vi "ta_calc_diff.vi"(0 "data in":dbl[][](array[numeric]), 5 "anisotropy input":T1, 9 "ref in":dbl[][](array[numeric]), 11 "Algorithm":T2=3 items=["<(S*-S)/S>/ln(10)", "<S*/S>-1", "<S*/PD*>/<S/PD>", "<S*/Sref*>/<S/Sref>", "<S*/Sref*/PD*>/<S/Sref>", "<S*/Sref*>/<S/Sref>_alt", "MA/r", "MA/r Sagnac", "FROG"], 12 "PD values in":dbl[][](array[numeric])) -> (1 "pumped std":dbl[](array[numeric]), 2 "anisotropy":T1, 3 "unpumped std":dbl[](array[numeric]), 4 "pumped":dbl[](array[numeric]), 6 "unpumped":dbl[](array[numeric]), 8 "diff std":dbl[](array[numeric]), 10 "diff":dbl[](array[numeric]), 14 "ref std":dbl[](array[numeric]), 15 "ref mean":dbl[](array[numeric]))   [LabVIEW 2019]
uses:
  data_algorithm.ctl
  <vilib>/Analysis/baseanly.llb/Mean (DBL).vi
  <vilib>/Analysis/NI_AALBase.lvlib
panel:
  out "size data":i32[](array[numeric])
  out "size ref":i32[](array[numeric])
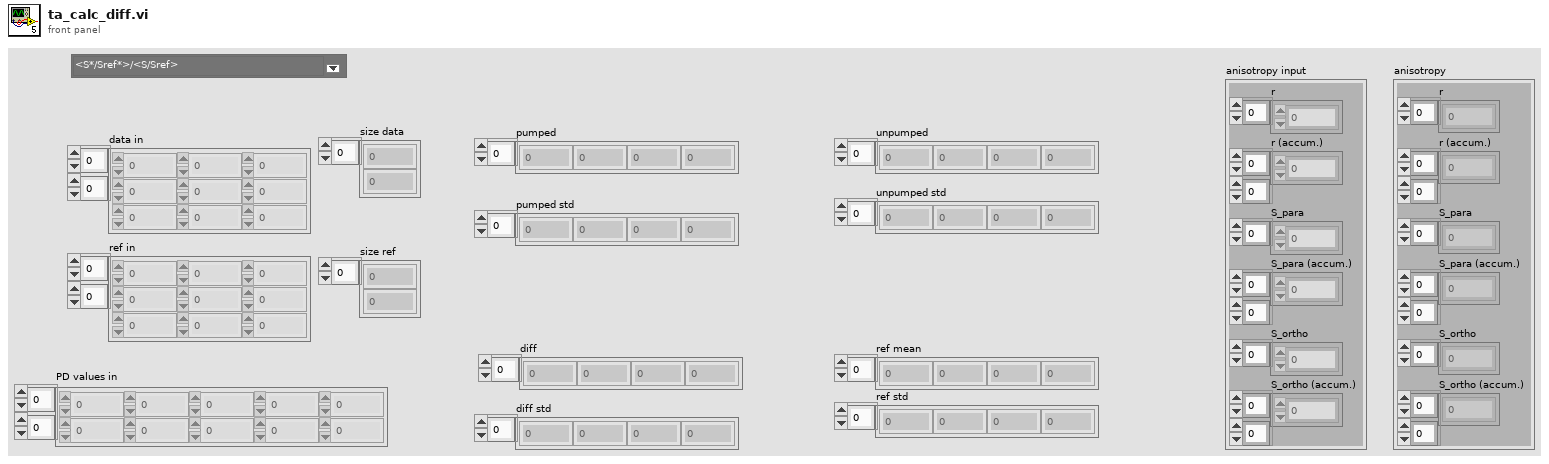
[diagram p1: front panel]
types:
  T1 = cluster{"r":dbl[], "r (accum.)":dbl[][], "S_para":dbl[], "S_para (accum.)":dbl[][], "S_ortho":dbl[], "S_ortho (accum.)":dbl[][]}
  T2 = typedef "data_algorithm.ctl" = u16
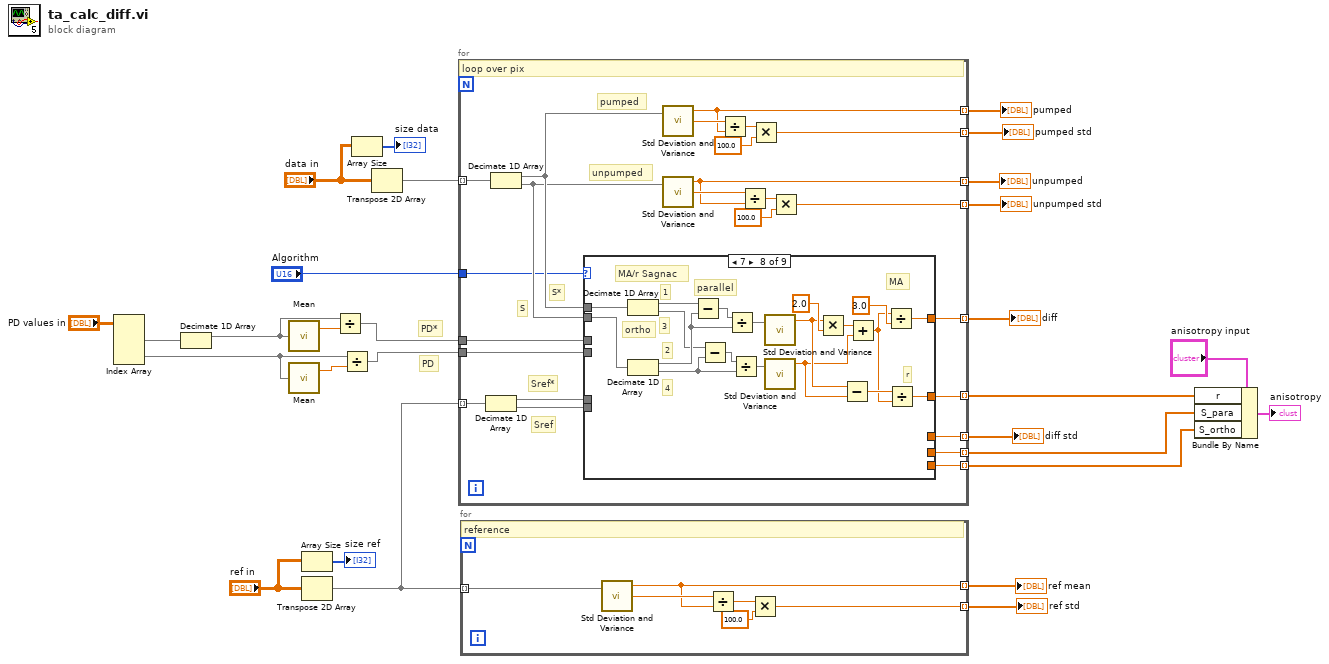
[diagram p0: block diagram]
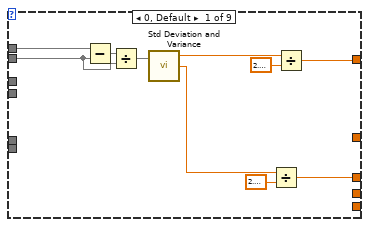
[diagram p2: hidden frame]
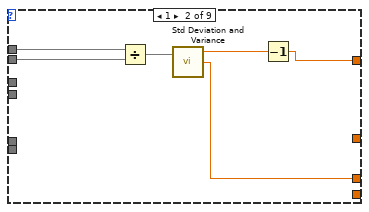
[diagram p3: hidden frame]
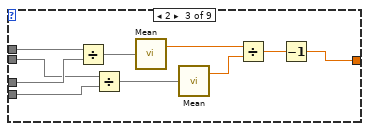
[diagram p4: hidden frame]
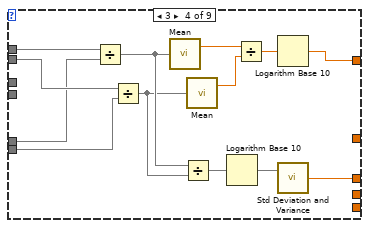
[diagram p5: hidden frame]
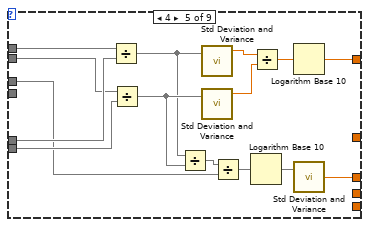
[diagram p6: hidden frame]
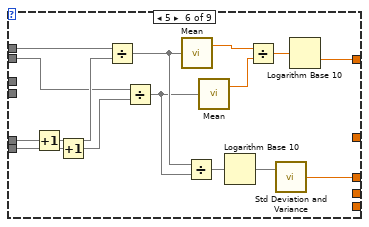
[diagram p7: hidden frame]
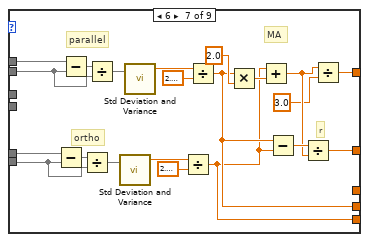
[diagram p8: hidden frame]
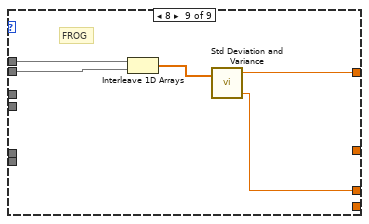
[diagram p9: hidden frame]
diagram:
  # "PD"
  # "PD*"
  n1 = Index Array(array="PD values in") -> (element #1=w8:dbl[], element #2=w11:dbl[])  [unwired: 4 in]
  n2 = Decimate 1D Array(w8) -> (w7:dbl[])  [unwired: 1 out]
  n3 = call-poly <vilib>:"Mean.vi"("X"=w7) -> ("mean"=w12:dbl)  [unwired: 1 out]
  n4 = call-poly <vilib>:"Mean.vi"("X"=w11) -> ("mean"=w10:dbl)  [unwired: 1 out]
  n5 = Array Size(array="ref in") -> (size(s)=→"size ref":i32[])
  n6 = Transpose 2D Array(2D array="ref in") -> (transposed array=w16:dbl[][])
  n7 = Divide(x=w7, y=w12) -> (x/y=w13:dbl[])
  n8 = Divide(x=w11, y=w10) -> (x/y=w9:dbl[])
  n9 = Array Size(array="data in") -> (size(s)=→"size data":i32[])
  n10 = Transpose 2D Array(2D array="data in") -> (transposed array=w22:dbl[][])
  n11 = for {
    tunnel: w22 -> [w50] mode=indexing
    tunnel: [w41] -> w28 mode=indexing
    tunnel: [w48] -> w27 mode=indexing
    tunnel: [w45] -> w20 mode=indexing
    tunnel: [w40] -> w19 mode=indexing
    tunnel: "Algorithm" -> [w39]
    tunnel: [w38] -> w17 mode=indexing
    tunnel: w13 -> [w33]
    tunnel: w9 -> [w37]
    tunnel: w16 -> [w36] mode=indexing
    tunnel: [w32] -> w6 mode=indexing
    tunnel: [w31] -> w4 mode=indexing
    tunnel: [w30] -> w3 mode=indexing
    tunnel: [w29] -> w2 mode=indexing
    # "Sref"
    # "Sref*"
    # "S"
    # "S*"
    # "unpumped"
    # "pumped"
    # "loop over pix"
    n12 = Decimate 1D Array(w36) -> (w35:dbl[], w34:dbl[])
    n13 = Decimate 1D Array(w50) -> (w52:dbl[], w51:dbl[])
    n14 = case shown="7" w39 {
      tunnel: w52 -> [w62 w68 w78 w91 w104 w115 w136 w161 w165]
      tunnel: w51 -> [w61 w67 w76 w90 w102 w114 w130 w160 w164]
      tunnel: [w56 w66 w69 w85 w105 w116 w125 w149 w163] -> w38
      tunnel: w33 -> [_ _ w77 _ w93 _ _ _ _]
      tunnel: w37 -> [_ _ w75 _ _ _ _ _ _]
      tunnel: w35 -> [_ _ _ w84 w103 w113 w135 _ _]
      tunnel: w34 -> [_ _ _ w89 w101 w112 w129 _ _]
      tunnel: [w53 w63 _ w79 w96 w107 _ _ w162] -> w32
      tunnel: [_ _ _ _ _ _ w127 w144 _] -> w31
      tunnel: [_ _ _ _ _ _ w123 _ _] -> w30
      tunnel: [_ _ _ _ _ _ w122 _ _] -> w29
      frame 0, Default {
        n15 = Subtract(x=w62, y=w61) -> (x-y=w57:dbl[])
        n16 = Divide(x=w57, y=w61) -> (x/y=w58:dbl[])
        n17 = call <vilib>:"Std Deviation and Variance.vi"("X"=w58) -> ("mean"=w59:dbl, "standard deviation"=w54:dbl)  [unwired: 1 in, 1 out]
        n18 = Divide(x=w54, y=2.302585092994046) -> (x/y=w53:dbl)
        n19 = Divide(x=w59, y=2.302585092994046) -> (x/y=w56:dbl)
      }
      frame 1 {
        n20 = Divide(x=w68, y=w67) -> (x/y=w65:dbl[])
        n21 = call <vilib>:"Std Deviation and Variance.vi"("X"=w65) -> ("mean"=w64:dbl, "standard deviation"=w63:dbl)  [unwired: 1 in, 1 out]
        n22 = Decrement(x=w64) -> (x-1=w66:dbl)
      }
      frame 2 {
        n23 = Divide(x=w78, y=w77) -> (x/y=w74:dbl[])
        n24 = Divide(x=w76, y=w75) -> (x/y=w73:dbl[])
        n25 = call-poly <vilib>:"Mean.vi"("X"=w74) -> ("mean"=w72:dbl)  [unwired: 1 out]
        n26 = call-poly <vilib>:"Mean.vi"("X"=w73) -> ("mean"=w71:dbl)  [unwired: 1 out]
        n27 = Divide(x=w72, y=w71) -> (x/y=w70:dbl)
        n28 = Decrement(x=w70) -> (x-1=w69:dbl)
      }
      frame 3 {
        n29 = Divide(x=w91, y=w84) -> (x/y=w83:dbl[])
        n30 = Divide(x=w90, y=w89) -> (x/y=w82:dbl[])
        n31 = call-poly <vilib>:"Mean.vi"("X"=w83) -> ("mean"=w88:dbl)  [unwired: 1 out]
        n32 = Divide(x=w83, y=w82) -> (x/y=w81:dbl[])
        n33 = call-poly <vilib>:"Mean.vi"("X"=w82) -> ("mean"=w87:dbl)  [unwired: 1 out]
        n34 = Logarithm Base 10(1:w81) -> (0:w80:dbl[])
        n35 = Divide(x=w88, y=w87) -> (x/y=w86:dbl)
        n36 = Logarithm Base 10(1:w86) -> (0:w85:dbl)
        n37 = call <vilib>:"Std Deviation and Variance.vi"("X"=w80) -> ("standard deviation"=w79:dbl)  [unwired: 1 in, 2 out]
      }
      frame 4 {
        n38 = Divide(x=w104, y=w103) -> (x/y=w95:dbl[])
        n39 = Divide(x=w102, y=w101) -> (x/y=w98:dbl[])
        n40 = Divide(x=w95, y=w98) -> (x/y=w94:dbl[])
        n41 = call <vilib>:"Std Deviation and Variance.vi"("X"=w95) -> ("mean"=w100:dbl)  [unwired: 1 in, 2 out]
        n42 = call <vilib>:"Std Deviation and Variance.vi"("X"=w98) -> ("mean"=w99:dbl)  [unwired: 1 in, 2 out]
        n43 = Divide(x=w94, y=w93) -> (x/y=w92:dbl[])
        n44 = Logarithm Base 10(1:w92) -> (0:w97:dbl[])
        n45 = Divide(x=w100, y=w99) -> (x/y=w106:dbl)
        n46 = Logarithm Base 10(1:w106) -> (0:w105:dbl)
        n47 = call <vilib>:"Std Deviation and Variance.vi"("X"=w97) -> ("standard deviation"=w96:dbl)  [unwired: 1 in, 2 out]
      }
      frame 5 {
        n48 = Increment(x=w113) -> (x+1=w120:dbl[])
        n49 = Increment(x=w112) -> (x+1=w121:dbl[])
        n50 = Divide(x=w115, y=w120) -> (x/y=w111:dbl[])
        n51 = Divide(x=w114, y=w121) -> (x/y=w110:dbl[])
        n52 = call-poly <vilib>:"Mean.vi"("X"=w111) -> ("mean"=w117:dbl)  [unwired: 1 out]
        n53 = Divide(x=w111, y=w110) -> (x/y=w109:dbl[])
        n54 = call-poly <vilib>:"Mean.vi"("X"=w110) -> ("mean"=w118:dbl)  [unwired: 1 out]
        n55 = Logarithm Base 10(1:w109) -> (0:w108:dbl[])
        n56 = Divide(x=w117, y=w118) -> (x/y=w119:dbl)
        n57 = call <vilib>:"Std Deviation and Variance.vi"("X"=w108) -> ("standard deviation"=w107:dbl)  [unwired: 1 in, 2 out]
        n58 = Logarithm Base 10(1:w119) -> (0:w116:dbl)
      }
      frame 6 {
        # "r"
        # "ortho"
        # "parallel"
        # "MA"
        n59 = Subtract(x=w135, y=w129) -> (x-y=w137:dbl[])
        n60 = Subtract(x=w136, y=w130) -> (x-y=w140:dbl[])
        n61 = Divide(x=w137, y=w129) -> (x/y=w131:dbl[])
        n62 = Divide(x=w140, y=w130) -> (x/y=w132:dbl[])
        n63 = call <vilib>:"Std Deviation and Variance.vi"("X"=w131) -> ("mean"=w138:dbl)  [unwired: 1 in, 2 out]
        n64 = call <vilib>:"Std Deviation and Variance.vi"("X"=w132) -> ("mean"=w141:dbl)  [unwired: 1 in, 2 out]
        n65 = Divide(x=w138, y=2.302585092994046) -> (x/y=w122:dbl)
        n66 = Divide(x=w141, y=2.302585092994046) -> (x/y=w123:dbl)
        n67 = Multiply(x=w123, y=2.0) -> (x*y=w133:dbl)
        n68 = Add(x=w122, y=w133) -> (x+y=w126:dbl)
        n69 = Subtract(x=w123, y=w122) -> (x-y=w128:dbl)
        n70 = Divide(x=w128, y=w126) -> (x/y=w127:dbl)
        n71 = Divide(x=w126, y=3.0) -> (x/y=w125:dbl)
      }
      frame 7 {
        # "ortho"
        # "parallel"
        # "r"
        # "MA"
        # "4"
        # "2"
        # "3"
        # "1"
        # "MA/r Sagnac"
        n72 = Decimate 1D Array(w161) -> (w159:dbl[], w155:dbl[])
        n73 = Decimate 1D Array(w160) -> (w157:dbl[], w143:dbl[])
        n74 = Subtract(x=w159, y=w157) -> (x-y=w158:dbl[])
        n75 = Subtract(x=w155, y=w143) -> (x-y=w154:dbl[])
        n76 = Divide(x=w158, y=w157) -> (x/y=w156:dbl[])
        n77 = Divide(x=w154, y=w143) -> (x/y=w153:dbl[])
        n78 = call <vilib>:"Std Deviation and Variance.vi"("X"=w156) -> ("mean"=w148:dbl)  [unwired: 1 in, 2 out]
        n79 = call <vilib>:"Std Deviation and Variance.vi"("X"=w153) -> ("mean"=w147:dbl)  [unwired: 1 in, 2 out]
        n80 = Multiply(x=w148, y=2.0) -> (x*y=w151:dbl)
        n81 = Subtract(x=w148, y=w147) -> (x-y=w146:dbl)
        n82 = Add(x=w151, y=w147) -> (x+y=w145:dbl)
        n83 = Divide(x=w145, y=3.0) -> (x/y=w149:dbl)
        n84 = Divide(x=w146, y=w145) -> (x/y=w144:dbl)
      }
      frame 8 {
        # "FROG"
        n85 = Interleave 1D Arrays(w165, w164) -> (w166:dbl[])
        n86 = call <vilib>:"Std Deviation and Variance.vi"("X"=w166) -> ("mean"=w163:dbl, "variance"=w162:dbl)  [unwired: 1 in, 1 out]
      }
    }
    n87 = call <vilib>:"Std Deviation and Variance.vi"("X"=w52) -> ("mean"=w48:dbl, "standard deviation"=w49:dbl)  [unwired: 1 in, 1 out]
    n88 = call <vilib>:"Std Deviation and Variance.vi"("X"=w51) -> ("mean"=w41:dbl, "standard deviation"=w42:dbl)  [unwired: 1 in, 1 out]
    n89 = Divide(x=w49, y=w48) -> (x/y=w47:dbl)
    n90 = Divide(x=w42, y=w41) -> (x/y=w44:dbl)
    n91 = Multiply(x=w47, y=100.0) -> (x*y=w45:dbl)
    n92 = Multiply(x=w44, y=100.0) -> (x*y=w40:dbl)
  }
  "diff" <- w17
  "unpumped" <- w28
  "pumped" <- w27
  "pumped std" <- w20
  "unpumped std" <- w19
  "diff std" <- w6
  n93 = for {
    tunnel: w16 -> [w172] mode=indexing
    tunnel: [w170] -> w26 mode=indexing
    tunnel: [w167] -> w21 mode=indexing
    # "reference"
    n94 = call <vilib>:"Std Deviation and Variance.vi"("X"=w172) -> ("mean"=w170:dbl, "standard deviation"=w171:dbl)  [unwired: 1 in, 1 out]
    n95 = Divide(x=w171, y=w170) -> (x/y=w169:dbl)
    n96 = Multiply(x=w169, y=100.0) -> (x*y=w167:dbl)
  }
  "ref mean" <- w26
  "ref std" <- w21
  n97 = Bundle By Name(cluster="anisotropy input", "r"=w4, "S_para"=w3, "S_ortho"=w2) -> (→"anisotropy":T1)
